vi "Disabled.vi"(7 "Robot Mode":T2, 10 "Match Info":T1={"Autonomous Elapsed Seconds"=0.0, "TeleOp Elapsed Seconds"=0.0, "Disabled Elapsed Seconds"=0.0, "Visited Autonomous"=FALSE, "Visited TeleOp"=FALSE, "Visited Disabled"=FALSE, "Autonomous Settings"={"Autonomous Style"=enum."Independent", "VI Refnum"=refnum}}, 11 "Call Context":T3) -> ()   [LabVIEW 2011]
doc: "This VI is called each time a disabled packet is received from the DS. It is often used to prepare for the next robot mode, to calibrate sensors, etc."
uses:
  <vilib>/Rock Robotics/WPI/DriverStation/WPI_DriverStationDerivedRobotMode.ctl
  <vilib>/Rock Robotics/WPI/DriverStation/WPI_DriverStationRobotMode.ctl
  <vilib>/Rock Robotics/WPI/DriverStation/WPI_DriverStationMatch Info.ctl
  <vilib>/Rock Robotics/WPI/DriverStation/DriverStationLCD/WPI_DriverStationLCDLCDLine.ctl
  Robot Global Data.vi
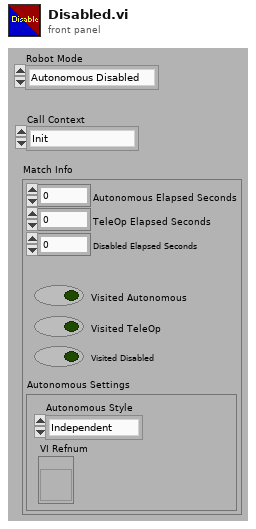
[diagram p1: front panel]
types:
  T1 = typedef "WPI_DriverStationMatch Info.ctl" = cluster{"Autonomous Elapsed Seconds":dbl, "TeleOp Elapsed Seconds":dbl, "Disabled Elapsed Seconds":dbl, "Visited Autonomous":bool, "Visited TeleOp":bool, "Visited Disabled":bool, "Autonomous Settings":cluster{"Autonomous Style":enum16{"Iterative", "Independent"}, "VI Refnum":refnum<vi>}}
  T2 = typedef "WPI_DriverStationRobotMode.ctl" = enum16{"Autonomous Disabled", "Autonomous Enabled", "Teleop Disabled", "Teleop Enabled", "Timeout", "Finish"}
  T3 = typedef "WPI_DriverStationDerivedRobotMode.ctl" = enum16{"Init", "Execute", "Stop"}
  T4 = typedef "WPI_DriverStationLCDLCDLine.ctl" = enum16{"Main - Line 1", "User - Line 2", "User - Line 3", "User - Line 4", "User - Line 5", "User - Line 6"}
  T5 = typedef "WPI_MotorControlDeviceRef.ctl" = cluster{"DeviceStatus":errorcluster, "Type":enum16{"PWM", "CAN"}, "PWM":cluster{"Digital Module":T6, "PWM Channel":T7, "DeadBand":T8}, "CAN":cluster{"Device Number":u8, "Control Mode":T9, "Semaphore":T10, "Max Vout":dbl}, "Invert":bool, "TransformRef":T11, "InvTransformRef":T11}
  T6 = typedef "FPGA_TypedefDigitalModule.ctl" = enum16{"Digital Module 1", "Digital Module 2"}
  T7 = typedef "FPGA_DIOPWMChannel.ctl" = enum8{"PWM 1", "PWM 2", "PWM 3", "PWM 4", "PWM 5", "PWM 6", "PWM 7", "PWM 8", "PWM 9", "PWM 10", "Invalid"}
  T8 = typedef "WPI_PWMDeadband.ctl" = cluster{"Name":string, "maxPositivePwm":i32, "minPositivePwm":i32, "centerPwm":i32, "maxNegativePwm":i32, "minNegativePwm":i32, "angularRange":u16}
  T9 = typedef "WPI_CANJaguar_ControlMode.ctl" = enum8{"Percent VBus", "Current", "Speed", "Position", "Voltage"}
  T10 = typedef "Semaphore RefNum" = refnum<k1>
  T11 = typedef "WPI_PWMTransform_ConPane.ctl" = refnum<vi>
  T12 = typedef "WPI_JoystickDevRef.ctl" = cluster{"Device":T13}
  T13 = typedef "WPI_JoystickDeviceEnum.ctl" = enum16{"USB 1", "USB 2", "USB 3", "USB 4", "Kinect 1", "Kinect 2"}
  T14 = typedef "WPI_JoystickButtonState.ctl" = cluster{"Button 1":bool, "Button 2":bool, "Button 3":bool, "Button 4":bool, "Button 5":bool, "Button 6":bool, "Button 7":bool, "Button 8":bool, "Button 9":bool, "Button 10":bool, "Button 11":bool, "Button 12":bool}
  T15 = typedef "WPI_ServoDeviceRef.ctl" = cluster{"DeviceStatus":errorcluster, "Digital Module":T6, "PWM Channel":T7, "DeadBand":T8}
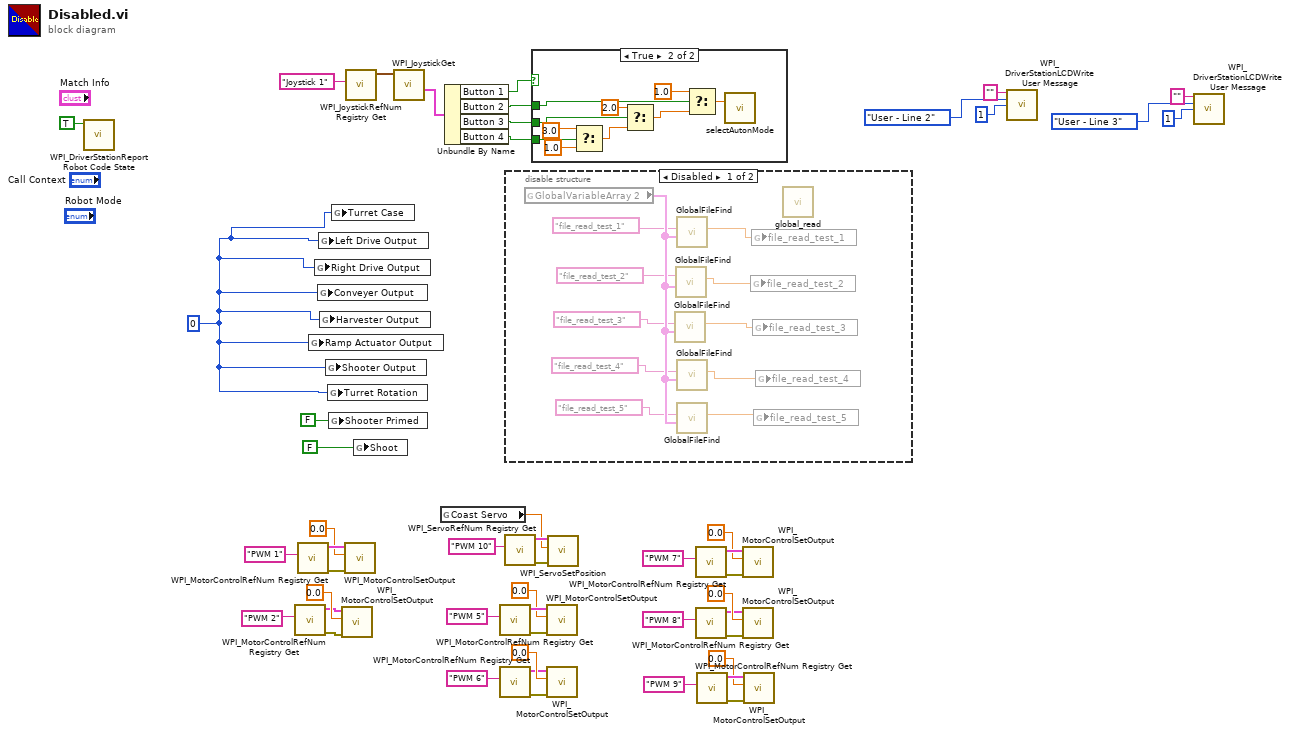
[diagram p0: block diagram]
diagram:
  w18 = 0
  n1 = call <vilib>:"WPI_DriverStationReport Robot Code State.vi"("Disabled"=TRUE ("Autonomous")) -> ()  [unwired: 10 in, 1 out]
  n2 = call <vilib>:"WPI_MotorControlRefNum Registry Get.vi"("refnum name"="PWM 2") -> ("error out"=w42:errorcluster, "MotorControlDevRef"=w41:T5)  [unwired: 9 in]
  n3 = call <vilib>:"WPI_MotorControlRefNum Registry Get.vi"("refnum name"="PWM 1") -> ("error out"=w47:errorcluster, "MotorControlDevRef"=w48:T5)  [unwired: 9 in]
  n4 = global write "Robot Global Data.vi" "Ramp Actuator Output"(w18) -> ()
  n5 = global write "Robot Global Data.vi" "Right Drive Output"(w18) -> ()
  n6 = global write "Robot Global Data.vi" "Conveyer Output"(w18) -> ()
  n7 = global write "Robot Global Data.vi" "Left Drive Output"(w18) -> ()
  n8 = global write "Robot Global Data.vi" "Harvester Output"(w18) -> ()
  n9 = global write "Robot Global Data.vi" "Shooter Output"(w18) -> ()
  n10 = global write "Robot Global Data.vi" "Turret Rotation"(w18) -> ()
  n11 = global write "Robot Global Data.vi" "Shooter Primed"(FALSE ("Shooter Primed")) -> ()
  n12 = global write "Robot Global Data.vi" "Turret Case"(w18) -> ()
  n13 = call <vilib>:"WPI_MotorControlSetOutput.vi"("error in (no error)"=w42, "Output"=0.0, "MotorControlDevRef"=w41) -> ()  [unwired: 7 in, 2 out]
  n14 = call <vilib>:"WPI_MotorControlSetOutput.vi"("error in (no error)"=w47, "Output"=0.0, "MotorControlDevRef"=w48) -> ()  [unwired: 7 in, 2 out]
  n15 = call <vilib>:"WPI_JoystickRefNum Registry Get.vi"("refnum name"="Joystick 1") -> ("JoystickDevRef"=w16:T12)  [unwired: 9 in, 1 out]
  n16 = global write "Robot Global Data.vi" "Shoot"(FALSE ("Shooter Primed")) -> ()
  n17 = call <vilib>:"WPI_JoystickGet.vi"("JoystickDevRef"=w16) -> ("Buttons"=w15:T14)  [unwired: 4 in, 2 out]
  n18 = global read "Robot Global Data.vi" "Coast Servo"() -> (w2:dbl)
  n19 = Unbundle By Name(w15) -> ("Button 1"=w14:bool, "Button 2"=w13:bool, "Button 3"=w12:bool, "Button 4"=w11:bool)
  n20 = call <vilib>:"WPI_MotorControlRefNum Registry Get.vi"("refnum name"="PWM 5") -> ("error out"=w39:errorcluster, "MotorControlDevRef"=w40:T5)  [unwired: 9 in]
  n21 = call <vilib>:"WPI_MotorControlRefNum Registry Get.vi"("refnum name"="PWM 6") -> ("error out"=w34:errorcluster, "MotorControlDevRef"=w33:T5)  [unwired: 9 in]
  n22 = call <vilib>:"WPI_ServoRefNum Registry Get.vi"("refnum name"="PWM 10") -> ("error out"=w4:errorcluster, "ServoDeviceRef"=w3:T15)  [unwired: 9 in]
  n23 = disable-structure shown="Disabled" {
    frame Disabled {
      n24 = global read "Robot Global Data.vi" "GlobalVariableArray 2"() -> (w60:cluster{"name":string, "va;":dbl}[])
      n25 = call "GlobalFileFind.vi"("GlobalVariableArray 2"=w60, "VariableNameLookup"="file_read_test_3") -> ("VariableValueOut"=w51:dbl)  [unwired: 9 in]
      n26 = call "GlobalFileFind.vi"("GlobalVariableArray 2"=w60, "VariableNameLookup"="file_read_test_2") -> ("VariableValueOut"=w50:dbl)  [unwired: 9 in]
      n27 = call "GlobalFileFind.vi"("GlobalVariableArray 2"=w60, "VariableNameLookup"="file_read_test_1") -> ("VariableValueOut"=w54:dbl)  [unwired: 9 in]
      n28 = call "GlobalFileFind.vi"("GlobalVariableArray 2"=w60, "VariableNameLookup"="file_read_test_4") -> ("VariableValueOut"=w52:dbl)  [unwired: 9 in]
      n29 = call "GlobalFileFind.vi"("GlobalVariableArray 2"=w60, "VariableNameLookup"="file_read_test_5") -> ("VariableValueOut"=w53:dbl)  [unwired: 9 in]
      n30 = global write "Robot Global Data.vi" "file_read_test_2"(w50) -> ()
      n31 = global write "Robot Global Data.vi" "file_read_test_1"(w54) -> ()
      n32 = global write "Robot Global Data.vi" "file_read_test_3"(w51) -> ()
      n33 = global write "Robot Global Data.vi" "file_read_test_5"(w53) -> ()
      n34 = global write "Robot Global Data.vi" "file_read_test_4"(w52) -> ()
      n35 = call "global_read.vi"() -> ()  [unwired: 12 in]
    }
    frame Enabled {
    }
  }
  n36 = case shown="True" w14 {
    tunnel: w13 -> [_ w67]
    tunnel: w12 -> [_ w65]
    tunnel: w11 -> [_ w70]
    frame False {
    }
    frame True {
      n37 = Select(t=3.0, s=w70, f=1.0) -> (s? t:f=w63:dbl)
      n38 = Select(t=2.0, s=w65, f=w63) -> (s? t:f=w62:dbl)
      n39 = Select(t=1.0, s=w67, f=w62) -> (s? t:f=w61:dbl)
      n40 = call "selectAutonMode.vi"("Auton File"=w61) -> ()  [unwired: 2 in]
    }
  }
  n41 = call <vilib>:"WPI_MotorControlSetOutput.vi"("error in (no error)"=w39, "Output"=0.0, "MotorControlDevRef"=w40) -> ()  [unwired: 7 in, 2 out]
  n42 = call <vilib>:"WPI_MotorControlSetOutput.vi"("error in (no error)"=w34, "Output"=0.0, "MotorControlDevRef"=w33) -> ()  [unwired: 7 in, 2 out]
  n43 = call <vilib>:"WPI_ServoSetPosition.vi"("error in (no error)"=w4, "Position"=w2, "ServoDeviceRef"=w3) -> ()  [unwired: 7 in, 2 out]
  n44 = call <vilib>:"WPI_MotorControlRefNum Registry Get.vi"("refnum name"="PWM 7") -> ("error out"=w31:errorcluster, "MotorControlDevRef"=w32:T5)  [unwired: 9 in]
  n45 = call <vilib>:"WPI_MotorControlRefNum Registry Get.vi"("refnum name"="PWM 8") -> ("error out"=w26:errorcluster, "MotorControlDevRef"=w25:T5)  [unwired: 9 in]
  n46 = call <vilib>:"WPI_MotorControlRefNum Registry Get.vi"("refnum name"="PWM 9") -> ("error out"=w23:errorcluster, "MotorControlDevRef"=w24:T5)  [unwired: 9 in]
  n47 = call <vilib>:"WPI_MotorControlSetOutput.vi"("error in (no error)"=w31, "Output"=0.0, "MotorControlDevRef"=w32) -> ()  [unwired: 7 in, 2 out]
  n48 = call <vilib>:"WPI_MotorControlSetOutput.vi"("error in (no error)"=w26, "Output"=0.0, "MotorControlDevRef"=w25) -> ()  [unwired: 7 in, 2 out]
  n49 = call <vilib>:"WPI_MotorControlSetOutput.vi"("error in (no error)"=w23, "Output"=0.0, "MotorControlDevRef"=w24) -> ()  [unwired: 7 in, 2 out]
  n50 = call <vilib>:"WPI_DriverStationLCDWrite User Message.vi"("line text"="", "line"=WPI_DriverStationLCDLCDLine."User - Line 2", "starting column"=i8 1) -> ()  [unwired: 2 in, 11 out]
  n51 = call <vilib>:"WPI_DriverStationLCDWrite User Message.vi"("line text"="", "line"=WPI_DriverStationLCDLCDLine."User - Line 3", "starting column"=i8 1) -> ()  [unwired: 2 in, 11 out]
